vi "degrees to milliseconds.vi"(11 "Distance in feet wanted":dbl) -> (3 "milliseconds":dbl)   [LabVIEW 2017]
panel:
  # "Doesn't do anything right now"
  # "Actually, it does"
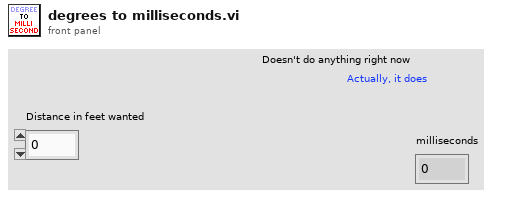
[diagram p1: front panel]
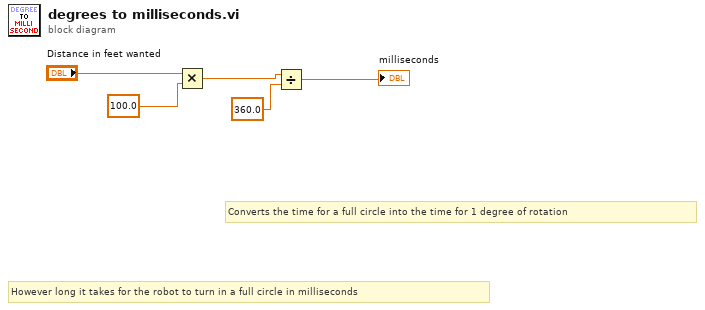
[diagram p0: block diagram]
diagram:
  # "Converts the time for a full circle into the time for 1 degree of rotation"
  # "However long it takes for the robot to turn in a full circle in milliseconds"
  n1 = Multiply(x="Distance in feet wanted", y=100.0) -> (x*y=w3:dbl)
  n2 = Divide(x=w3, y=360.0) -> (x/y=→"milliseconds":dbl)
